vi "Query - String - 1D.vi"(8 "error in":errorcluster, 10 "Query":string, 11 "Module ID":i32=-1) -> (0 "error out":errorcluster, 1 "Meta Data":variant, 2 "Return Data":string[](array[string]), 4 "Field Names":string[](array[string]))   [LabVIEW 2020, in "hse-db.lvlib" / "DB_CONNECTOR.lvlib"]
doc: "returns the first row\n\n____\nHAMPEL SOFTWARE ENGINEERING v1.4.0 (2023-12-19 09:52)"
uses:
  DB_CONNECTOR.lvlib
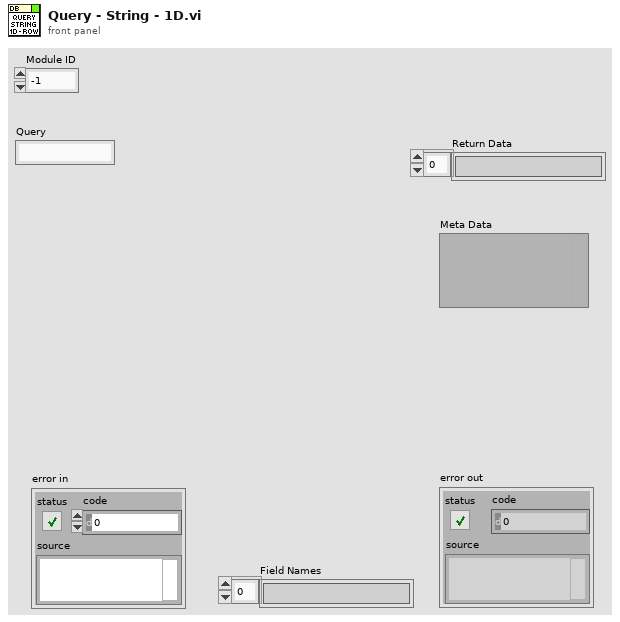
[diagram p1: front panel]
types:
  T1 = typedef "hse-db.lvlib/DB_CONNECTOR.lvlib/Query (Reply Payload)--cluster.ctl" = cluster{"Return Data":string[][], "Meta Data":variant, "Field Names":string[], "Query_error":errorcluster, "Module ID":i32}
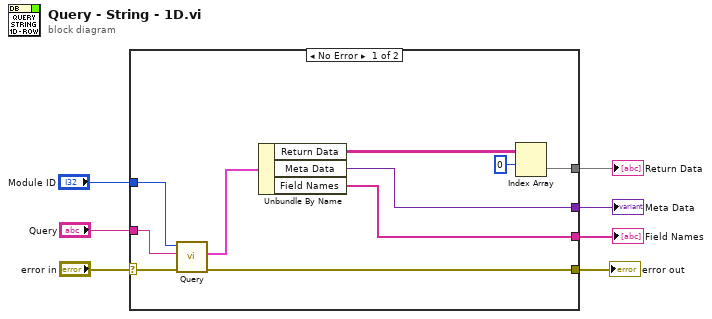
[diagram p0: block diagram]
diagram:
  n1 = case shown="No Error" "error in" {
    selector: "error in" -> [w12 w18]
    tunnel: [w8 w18] -> w6
    tunnel: "Query" -> [w11 _]
    tunnel: "Module ID" -> [w10 _]
    tunnel: [w16 _] -> w2
    tunnel: [w14 _] -> w3
    tunnel: [w13 _] -> w1
    frame No Error {
      n2 = call "Query.vi"("error in (no error)"=w12, "Query"=w11, "Module ID"=w10) -> ("error out"=w8:errorcluster, "Reply Payload"=w9:T1)  [unwired: 6 in, 1 out]
      n3 = Unbundle By Name(w9) -> ("Return Data"=w17:string[][], "Meta Data"=w16:variant, "Field Names"=w13:string[])
      n4 = Index Array(array=w17, index (row)=0) -> (element=w14:string[])  [unwired: 1 in]
    }
    frame Error {
    }
  }
  "error out" <- w6
  "Return Data" <- w3
  "Meta Data" <- w2
  "Field Names" <- w1
